vi "LVClass_WavefrontCorrectorSet get initial actuators specifications.vi"(0 "WavefrontCorrectorSet in":refnum<class "WavefrontCorrectorSet.lvclass">, 11 "error in (no error)":errorcluster) -> (4 "WavefrontCorrectorSet out":refnum<class "WavefrontCorrectorSet.lvclass">, 6 "Wavefront Corrector State":T1[](array[typedef]), 15 "error out":errorcluster)   [LabVIEW 2020, in "WavefrontCorrectorSet.lvclass"]
doc: "WavefrontCorrector constraints getter.\n\n--------------------------------------------------------------------------------\n\n<B>wavefrontcorrector_setIn </B> : WavefrontCorrectorSet object.\n<B>wavefrontcorrector_setOut </B> : WavefrontCorrectorSet object.\n<B>max </B> : WavefrontCorrector preferences : highest command value. See\n cWavefrontCorrector.\n<B>min </B> : WavefrontCorrector preferences : lowest command value. See\n cWavefrontCorrector.\n<B>validity </B> : WavefrontCorrector preferences : status. See cWavefrontCorrector.\n<B>position </B> : WavefrontCorrector preferences : fixed positions. See cWavefrontCorrector.\n<B>ErrorIn </B> : Error\n<B>ErrorOut </B> : Error\n\n--------------------------------------------------------------------------------"
uses:
  WavefrontCorrectorSet.lvclass
  Controls/Wavefront Corrector states - ONE.ctl
  WavefrontCorrectorSet.lvclass/WavefrontCorrectorSet.ctl
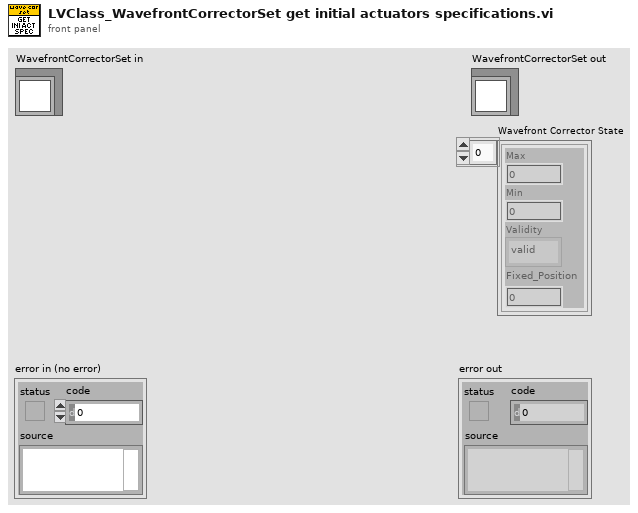
[diagram p1: front panel]
types:
  T1 = typedef "Wavefront Corrector states - ONE.ctl" = cluster{"Max":sgl, "Min":sgl, "Validity":enum16{"valid", "fixed", "invalid"}, "Fixed_Position":sgl}
  T2 = typedef "ClassID.ctl" = i64
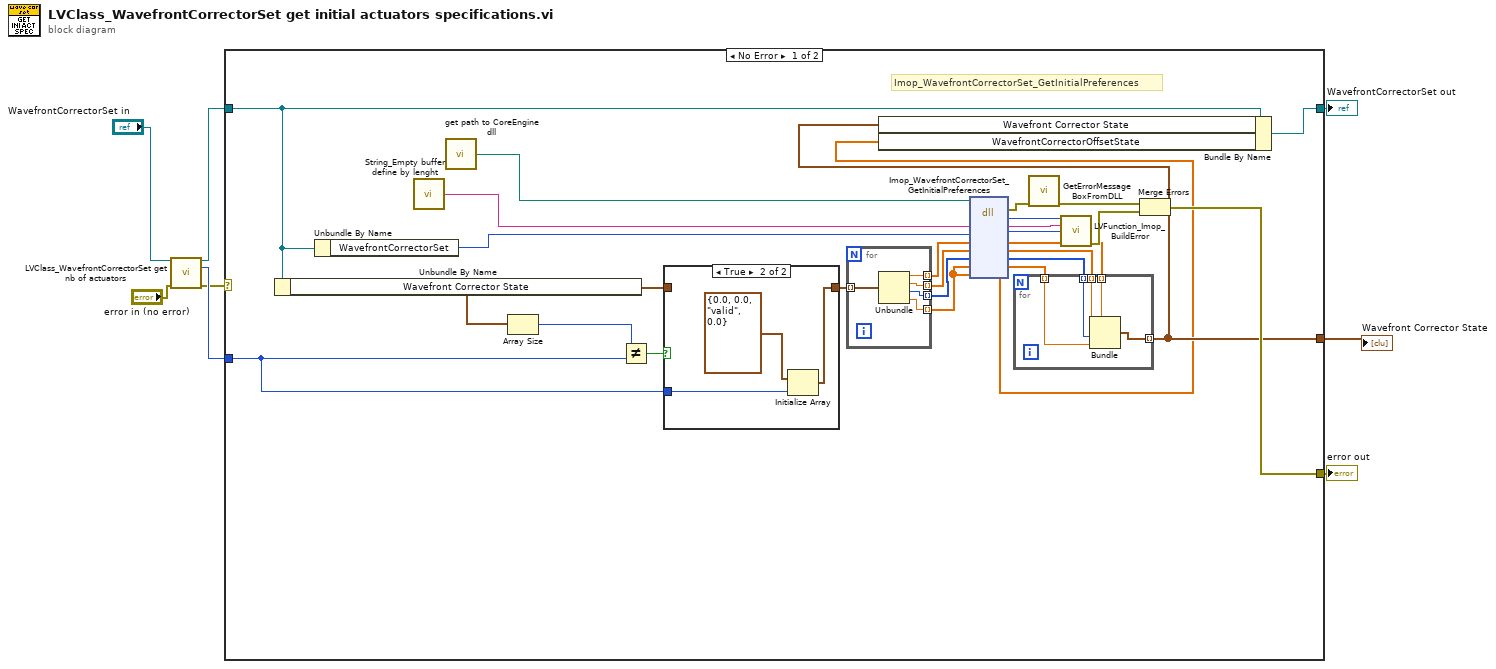
[diagram p0: block diagram]
diagram:
  n1 = call "LVClass_WavefrontCorrectorSet get nb of actuators.vi"("WavefrontCorrectorSet in"="WavefrontCorrectorSet in", "error in (no error)"="error in (no error)") -> ("WavefrontCorrectorSet out"=w2:refnum<class "WavefrontCorrectorSet.lvclass">, "ActuatorsNumber"=w6:i32, "error out"=w4:errorcluster)  [unwired: 11 in]
  n2 = case shown="No Error" w4 {
    selector: w4 -> [_ w51]
    tunnel: [w27 w51] -> w8
    tunnel: [w14 w50] -> w7
    tunnel: w2 -> [w15 w50]
    tunnel: w6 -> [w19 _]
    tunnel: [w12 _] -> w1
    frame No Error {
      # "Imop_WavefrontCorrectorSet_GetInitialPreferences"
      n3 = Unbundle By Name(w15) -> ("Wavefront Corrector State"=w20:T1[])
      n4 = Unbundle By Name(w15) -> ("WavefrontCorrectorSet"=w28:T2)
      n5 = call "String_Empty buffer define by lenght.vi"() -> ("Empty buffer"=w33:string)  [unwired: 1 in]
      n6 = call "get path to CoreEngine dll.vi"() -> ("path to wavekit library"=w32:path)  [unwired: 14 in, 1 out]
      n7 = Array Size(array=w20) -> (size(s)=w10:i32)
      n8 = Not Equal?(x=w10, y=w19) -> (x != y?=w22:bool)
      n9 = case shown="True" w22 {
        tunnel: [w41 w43] -> w21
        tunnel: w19 -> [_ w44]
        tunnel: w20 -> [w41 _]
        frame False {
        }
        frame True {
          n10 = Initialize Array(T1 {"Max"=0.0, "Min"=0.0, "Validity"=enum."valid", "Fixed_Position"=0.0} ("Actuator state"), w44) -> (w43:T1[])
        }
      }
      n11 = for {
        tunnel: w21 -> [w40] mode=indexing
        tunnel: [w39] -> w18 mode=indexing
        tunnel: [w38] -> w17 mode=indexing
        tunnel: [w37] -> w16 mode=indexing
        tunnel: [w36] -> w13 mode=indexing
        n12 = Unbundle(w40) -> ("Max"=w39:sgl, "Min"=w38:sgl, "Validity"=w37:enum16{"valid", "fixed", "invalid"}, "Fixed_Position"=w36:sgl)
      }
      n13 = dll-call lib="D:/soft/HASO_v3/C_interface/Sources/Build/vc100/Release/c_interface_vc100.dll" fn="Imop_WavefrontCorrectorSet_GetInitialPreferences"(path in=w32, "message"=w33, "WavefrontCorrectionSet"=w28, "Tab max"=w18, "tab min"=w17, "tab validity"=w16, "fixed_values"=w13, "init_positions"=w13) -> (error out=w31:errorcluster, "return type"=w35:i32, "message"=w34:string, "WavefrontCorrectionSet"=w9:i64, "Tab max"=w26:sgl[], "tab min"=w25:sgl[], "tab validity"=w24:i32[], "fixed_values"=w23:sgl[], "init_positions"=w11:sgl[])  [unwired: 2 in, 1 out]
      n14 = for {
        tunnel: w26 -> [w49] mode=indexing
        tunnel: w25 -> [w48] mode=indexing
        tunnel: w24 -> [w47] mode=indexing
        tunnel: w23 -> [w46] mode=indexing
        tunnel: [w45] -> w12 mode=indexing
        n15 = Bundle(w49, w48, w47, w46) -> (w45:cluster{sgl, sgl, i32, sgl})  [unwired: 1 in]
      }
      n16 = Bundle By Name(cluster=w15, "Wavefront Corrector State"=w12, "WavefrontCorrectorOffsetState"=w11) -> (w14:refnum<class "WavefrontCorrectorSet.lvclass">)
      n17 = call "GetErrorMessageBoxFromDLL.vi"("error IN"=w31) -> ("error OUT"=w30:errorcluster)  [unwired: 10 in]
      n18 = call "LVFunction_Imop_BuildError.vi"("code"=w35, "String to Prepend to source (\"\")"=w34, "Adresse"=w9) -> ("error out"=w29:errorcluster)  [unwired: 12 in]
      n19 = Merge Errors(w30, w29) -> (w27:errorcluster)
    }
    frame Error {
    }
  }
  "error out" <- w8
  "WavefrontCorrectorSet out" <- w7
  "Wavefront Corrector State" <- w1
